vi "convert.vi"(8 "error in (no error)":errorcluster, 10 "Input":dbl, 11 "ConvertROTRawToEngStrategy in":refnum<class "ConvertROTRawToEngStrategy.lvclass">) -> (0 "error out":errorcluster, 2 "Output":dbl, 3 "ConvertROTRawToEngStrategy out":refnum<class "ConvertROTRawToEngStrategy.lvclass">)   [LabVIEW 2015, in "ConvertROTRawToEngStrategy.lvclass"]
uses:
  ConvertROTRawToEngStrategy.lvclass
  ConvertROTRawToEngStrategy.lvclass/ConvertROTRawToEngStrategy.ctl
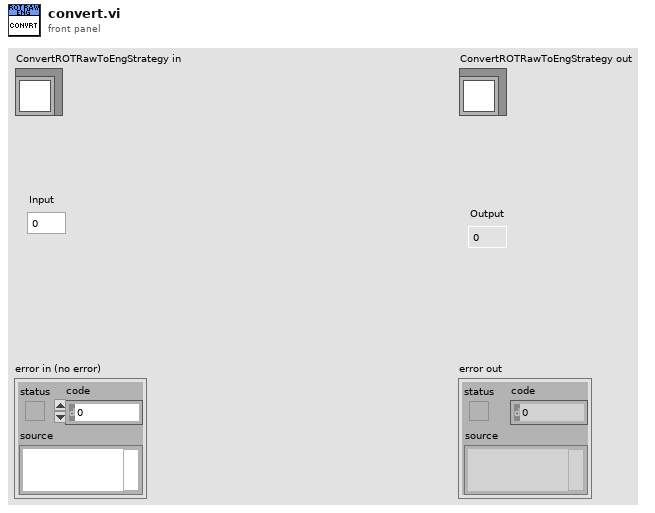
[diagram p1: front panel]
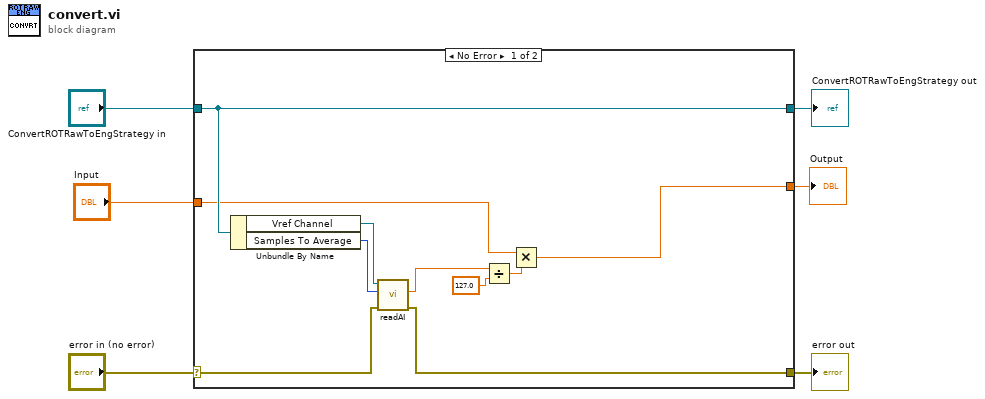
[diagram p0: block diagram]
diagram:
  n1 = case shown="No Error" "error in (no error)" {
    selector: "error in (no error)" -> [w11 w19]
    tunnel: [w7 w19] -> w5
    tunnel: [w14 w18] -> w3
    tunnel: "ConvertROTRawToEngStrategy in" -> [w14 w18]
    tunnel: "Input" -> [w9 w17]
    tunnel: [w8 w17] -> w1
    frame No Error {
      n2 = Unbundle By Name(w14) -> ("Vref Channel"=w12:refnum<k21>, "Samples To Average"=w13:i32)
      n3 = call "readAI.vi"("error in (no error)"=w11, "Samples To Read"=w13, "DAQ Channel To Read"=w12) -> ("error out"=w7:errorcluster, "Average"=w10:dbl)  [unwired: 6 in, 1 out]
      n4 = Divide(x=w10, y=127.0) -> (x/y=w16:dbl)
      n5 = Multiply(x=w9, y=w16) -> (x*y=w8:dbl)
    }
    frame Error {
    }
  }
  "error out" <- w5
  "ConvertROTRawToEngStrategy out" <- w3
  "Output" <- w1
